vi "Query the test reaults for the scanner box.vi"(0 "VISA resource name":refnum<visa-resource-name>, 5 "error in":errorcluster) -> (14 "VISA resource name out":refnum<visa-resource-name>, 15 "Test Results for 1ST":string, 16 "Test Results for 2ND":string, 17 "Test Results for 3RD":string, 18 "Test Results for 4TH":string, 19 "error out":errorcluster)   [LabVIEW 2011, in "GPT-9000.lvlib"]
uses:
  <instrlib>/GPT-9000/GPT-9000.lvlib
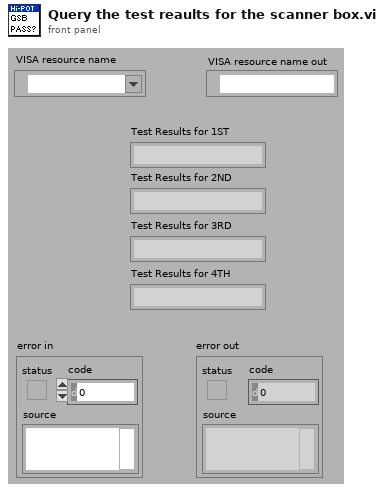
[diagram p1: front panel]
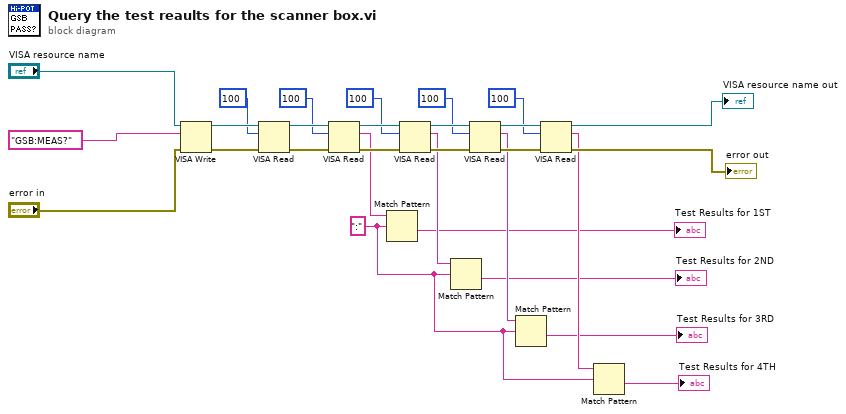
[diagram p0: block diagram]
diagram:
  w1 = ":" ("regular expression")
  n1 = VISA Write(VISA resource name="VISA resource name", write buffer="GSB:MEAS?", error in (no error)="error in") -> (VISA resource name out=w26:refnum<visa-resource-name>, error out=w21:errorcluster)  [unwired: 1 out]
  n2 = VISA Read(VISA resource name=w26, byte count=u32 100, error in (no error)=w21) -> (VISA resource name out=w25:refnum<visa-resource-name>, error out=w20:errorcluster)  [unwired: 2 out]
  n3 = VISA Read(VISA resource name=w25, byte count=u32 100, error in (no error)=w20) -> (VISA resource name out=w24:refnum<visa-resource-name>, read buffer=w9:string, error out=w19:errorcluster)  [unwired: 1 out]
  n4 = Match Pattern(string=w9, regular expression=w1) -> (after substring=→"Test Results for 1ST":string)  [unwired: 1 in, 3 out]
  n5 = VISA Read(VISA resource name=w24, byte count=u32 100, error in (no error)=w19) -> (VISA resource name out=w23:refnum<visa-resource-name>, read buffer=w8:string, error out=w18:errorcluster)  [unwired: 1 out]
  n6 = Match Pattern(string=w8, regular expression=w1) -> (after substring=→"Test Results for 2ND":string)  [unwired: 1 in, 3 out]
  n7 = VISA Read(VISA resource name=w23, byte count=u32 100, error in (no error)=w18) -> (VISA resource name out=w22:refnum<visa-resource-name>, read buffer=w7:string, error out=w17:errorcluster)  [unwired: 1 out]
  n8 = Match Pattern(string=w7, regular expression=w1) -> (after substring=→"Test Results for 3RD":string)  [unwired: 1 in, 3 out]
  n9 = VISA Read(VISA resource name=w22, byte count=u32 100, error in (no error)=w17) -> (VISA resource name out=→"VISA resource name out":refnum<visa-resource-name>, read buffer=w6:string, error out=→"error out":errorcluster)  [unwired: 1 out]
  n10 = Match Pattern(string=w6, regular expression=w1) -> (after substring=→"Test Results for 4TH":string)  [unwired: 1 in, 3 out]
